vi "Teleop.vi"(10 "Match Info":T1={"Autonomous Elapsed Seconds"=0.0, "TeleOp Elapsed Seconds"=0.0, "Disabled Elapsed Seconds"=0.0, "Visited Autonomous"=FALSE, "Visited TeleOp"=FALSE, "Visited Disabled"=FALSE, "Autonomous Settings"={"Autonomous Style"=enum."Independent", "VI Refnum"=refnum}}, 11 "Call Context":T2) -> ()   [LabVIEW 2020]
doc: "This VI is called for each TeleOp packet received from the DS where the robot is not disabled. It is often used to read from the joysticks and update I/O or to update setpoints for timed control loops. It should complete and return within 20 milliseconds or it may miss DS packets."
uses:
  <vilib>/Rock Robotics/WPI/DriverStation/WPI_DriverStationDerivedRobotMode.ctl
  <vilib>/Rock Robotics/WPI/DriverStation/WPI_DriverStationMatch Info.ctl
  <vilib>/Rock Robotics/WPI/Utilities/WPI_GetSetVariantRefNum.vi
  <vilib>/Rock Robotics/Network Tables/NT Write Boolean Array.vi
  <vilib>/Rock Robotics/Network Tables/NT Write Numeric Array.vi
  <vilib>/Rock Robotics/Network Tables/NT Read Boolean.vi
  <vilib>/Rock Robotics/Network Tables/NT Read Number.vi
  Robot Global Data.vi
panel:
  out "Sample Slider 0":dbl(slide) scale=0.0..5.0
  out "Sample Boolean 1":bool
  out "Sample Boolean 0":bool
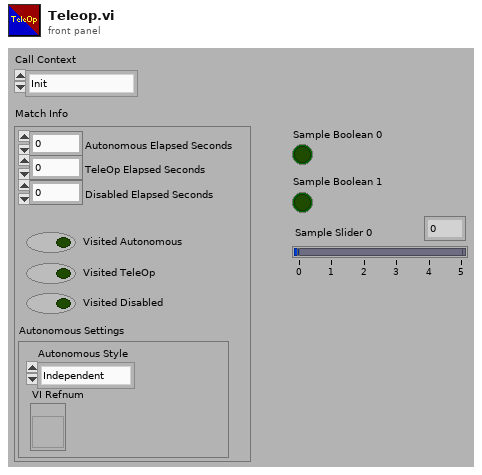
[diagram p1: front panel]
types:
  T1 = typedef "WPI_DriverStationMatch Info.ctl" = cluster{"Autonomous Elapsed Seconds":dbl, "TeleOp Elapsed Seconds":dbl, "Disabled Elapsed Seconds":dbl, "Visited Autonomous":bool, "Visited TeleOp":bool, "Visited Disabled":bool, "Autonomous Settings":cluster{"Autonomous Style":enum16{"Iterative", "Independent"}, "VI Refnum":refnum<vi>}}
  T2 = typedef "WPI_DriverStationDerivedRobotMode.ctl" = enum16{"Init", "Execute", "Stop"}
  T3 = typedef "WPI_JoystickDevRef.ctl" = cluster{"Device":T4}
  T4 = typedef "WPI_JoystickDeviceEnum.ctl" = enum16{"USB 0", "USB 1", "USB 2", "USB 3", "USB 4", "USB 5"}
  T5 = typedef "WPI_RobotDriveDevRef.ctl" = cluster{"DevStatus":errorcluster, "Motors[]":T6[], "Square Inputs":bool, "Max Output":dbl}
  T6 = typedef "WPI_MotorControlDeviceRef.ctl" = cluster{"DeviceStatus":errorcluster, "Type":T7, "PWM":cluster{"PWM Channel":T8, "DeadBand":T9}, "CAN":cluster{"Device Number":u8, "SetOutput VI Ref":variant, "GetOutput VI Ref":variant, "Enable VI Ref":variant, "Disable VI Ref":variant, "Data":variant}, "Invert":bool, "DIO PWM":cluster{"PWM \"Enable\" Channel":T8, "DIOChannel":T10, "PWM Rate":dbl}}
  T7 = typedef "WPI_MotorControlType.ctl" = enum16{"PWM", "CAN", "DIO PWM"}
  T8 = typedef "FPGA_DIOPWMChannel.ctl" = enum8{"PWM 0", "PWM 1", "PWM 2", "PWM 3", "PWM 4", "PWM 5", "PWM 6", "PWM 7", "PWM 8", "PWM 9", "PWM MXP 0", "PWM MXP 1", "PWM MXP 2", "PWM MXP 3", "PWM MXP 4", "PWM MXP 5", "PWM MXP 6", "PWM MXP 7", "PWM MXP 8", "PWM MXP 9", "Invalid"}
  T9 = typedef "WPI_PWMDeadband.ctl" = cluster{"Name":string, "maxPositivePwm":i32, "minPositivePwm":i32, "centerPwm":i32, "maxNegativePwm":i32, "minNegativePwm":i32, "angularRange":u16}
  T10 = typedef "FPGA_DIOChannel.ctl" = enum8{"DIO 0", "DIO 1", "DIO 2", "DIO 3", "DIO 4", "DIO 5", "DIO 6", "DIO 7", "DIO 8", "DIO 9", "DIO MXP 0", "DIO MXP 1", "DIO MXP 2", "DIO MXP 3", "DIO MXP 4", "DIO MXP 5", "DIO MXP 6", "DIO MXP 7", "DIO MXP 8", "DIO MXP 9", "DIO MXP 10", "DIO MXP 11", "DIO MXP 12", "DIO MXP 13", "DIO MXP 14", "DIO MXP 15", "SPI Port CS1", "SPI Port CS2", "SPI Port CS3", "SPI Port MISO", "SPI Port MOSI", "Invalid"}
  T11 = cluster{"Buttons[0]":bool, "Buttons[1]":bool, "Buttons[2]":bool, "Buttons[3]":bool, "Buttons[4]":bool, "Buttons[5]":bool, "Buttons[6]":bool, "Buttons[7]":bool, "Buttons[8]":bool}
  T12 = cluster{"Axes[0]":dbl, "Axes[1]":dbl, "Axes[2]":dbl, "Axes[3]":dbl, "Axes[4]":dbl, "Axes[5]":dbl, "Axes[6]":dbl, "Axes[7]":dbl, "Axes[8]":dbl}
  T13 = typedef "WPI_DigitalOutputDevRef.ctl" = cluster{"DIO Channel":T10, "DevStatus":errorcluster}
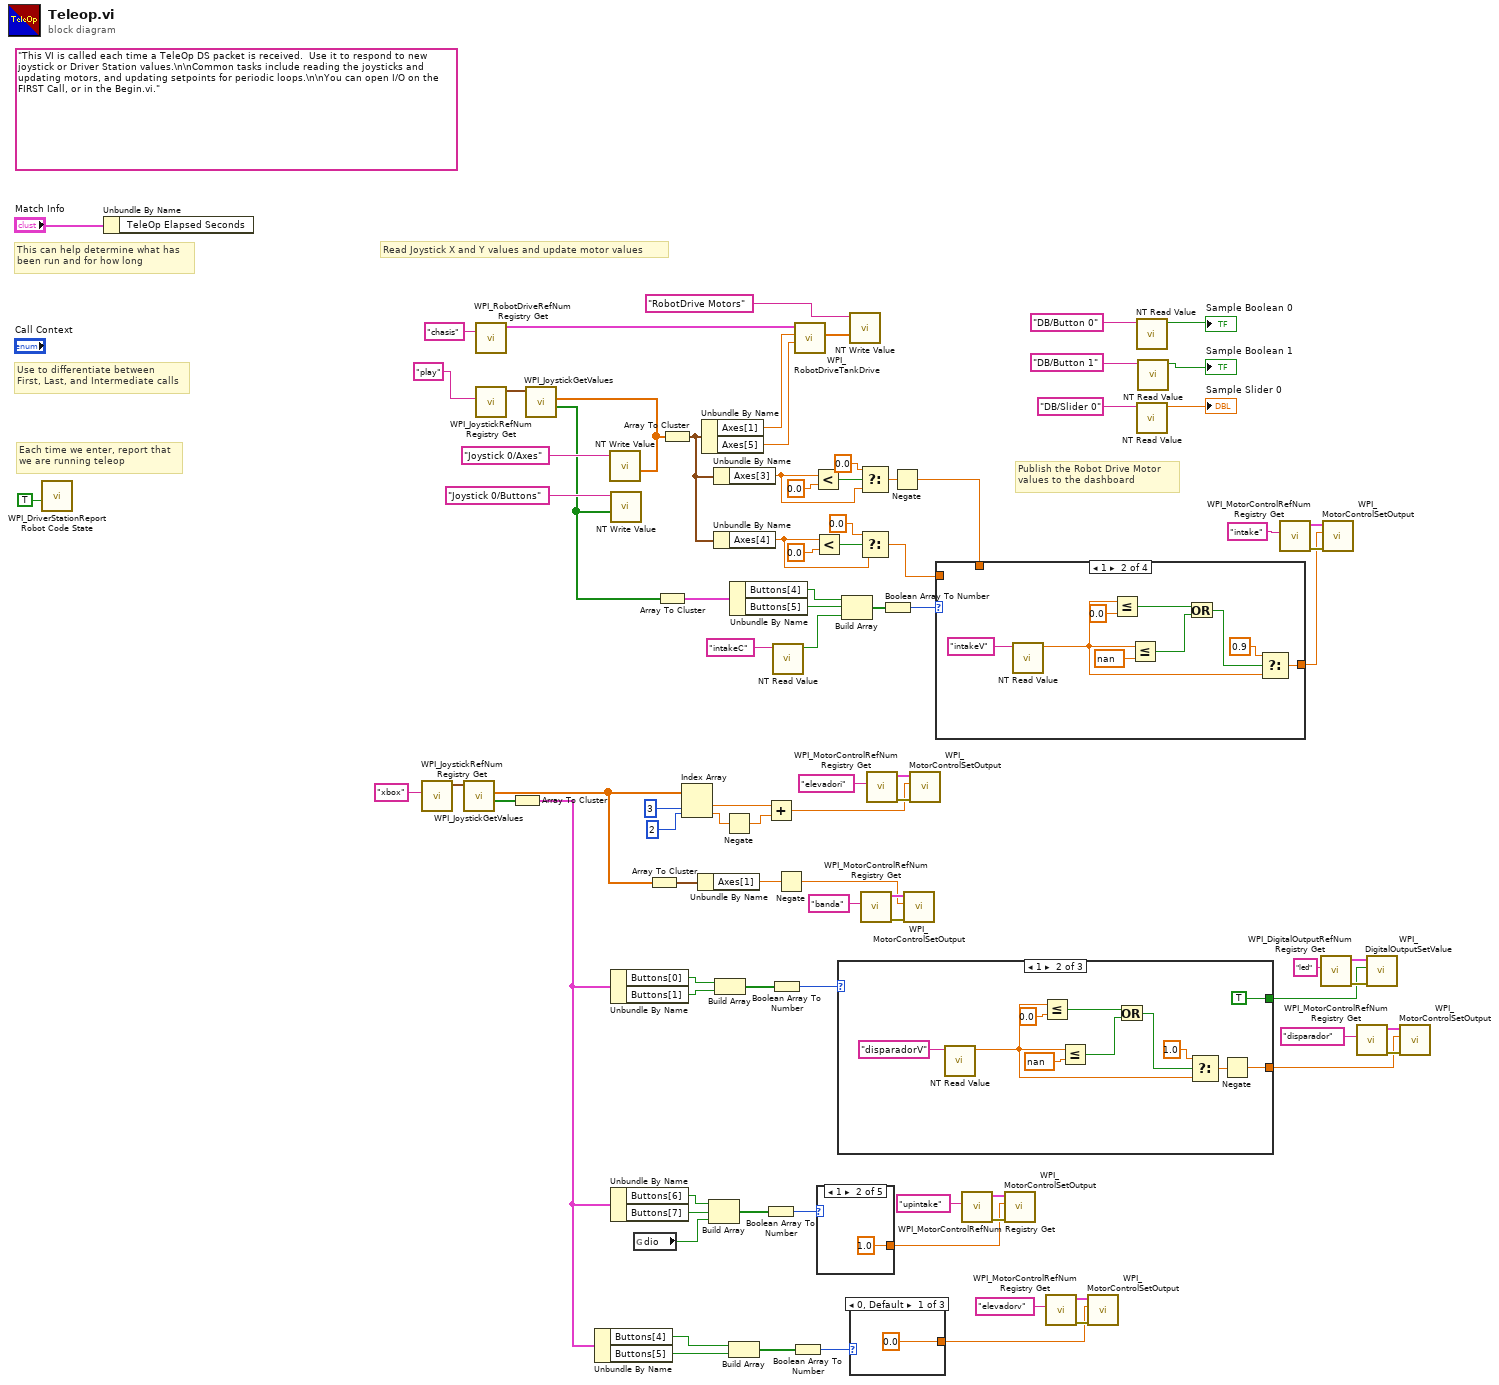
[diagram p0: block diagram]
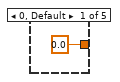
[diagram p2: hidden frame]
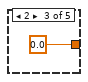
[diagram p3: hidden frame]
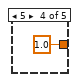
[diagram p4: hidden frame]
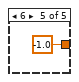
[diagram p5: hidden frame]
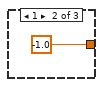
[diagram p6: hidden frame]
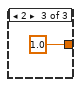
[diagram p7: hidden frame]
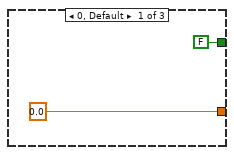
[diagram p8: hidden frame]
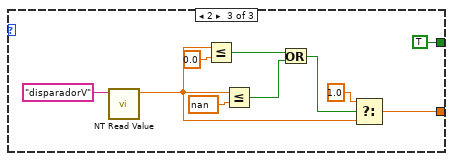
[diagram p9: hidden frame]
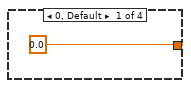
[diagram p10: hidden frame]
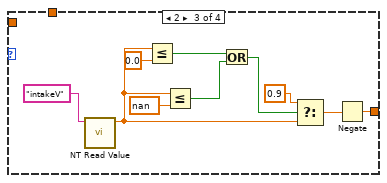
[diagram p11: hidden frame]
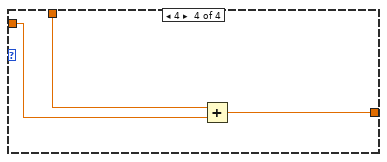
[diagram p12: hidden frame]
diagram:
  (unwired) "This VI is called each time a TeleOp DS packet is received.  Use it to respond to new joystick or Driver Station values.\n\nCommon tasks include reading the joysticks and updating motors, and updating setpoints for periodic loops.\n\nYou can open I/O on the FIRST Call, or in the Begin.vi."
  # "Publish the Robot Drive Motor\nvalues to the dashboard"
  # "Each time we enter, report that\nwe are running teleop"
  # "Use to differentiate between\nFirst, Last, and Intermediate calls"
  # "This can help determine what has\nbeen run and for how long"
  # "Read Joystick X and Y values and update motor values"
  n1 = call <vilib>:"WPI_DriverStationReport Robot Code State.vi"("TeleOp"=TRUE ("Autonomous")) -> ()  [unwired: 10 in, 1 out]
  n2 = Unbundle By Name("Match Info") -> ()  [unwired: 1 out]
  n3 = call <vilib>:"WPI_JoystickRefNum Registry Get.vi"("refnum name"="xbox") -> ("JoystickDevRef"=w73:T3)  [unwired: 1 in, 9 out]
  n4 = call <vilib>:"WPI_JoystickGetValues.vi"("JoystickDevRef"=w73) -> ("Buttons"=w58:bool[], "Axes"=w11:dbl[])  [unwired: 6 in, 3 out]
  n5 = call <vilib>:"WPI_RobotDriveRefNum Registry Get.vi"("refnum name"="chasis") -> ("RobotDriveDevRef"=w90:T5)  [unwired: 1 in, 9 out]
  n6 = call <vilib>:"WPI_JoystickRefNum Registry Get.vi"("refnum name"="play") -> ("JoystickDevRef"=w88:T3)  [unwired: 1 in, 9 out]
  n7 = Array To Cluster(array=w58) -> (cluster=w34:T11)
  n8 = call <vilib>:"WPI_JoystickGetValues.vi"("JoystickDevRef"=w88) -> ("Buttons"=w2:bool[], "Axes"=w37:dbl[])  [unwired: 6 in, 3 out]
  n9 = Unbundle By Name(w34) -> ("Buttons[4]"=w57:bool, "Buttons[5]"=w56:bool)
  n10 = call-poly <vilib>:"NT Write Value.vi"("Numeric Array"=w37, "Name"="Joystick 0/Axes") -> ()  [unwired: 9 in, 1 out]
  n11 = call-poly <vilib>:"NT Write Value.vi"("Boolean Array"=w2, "Name"="Joystick 0/Buttons") -> ()  [unwired: 9 in, 1 out]
  n12 = Unbundle By Name(w34) -> ("Buttons[0]"=w8:bool, "Buttons[1]"=w7:bool)
  n13 = Unbundle By Name(w34) -> ("Buttons[6]"=w48:bool, "Buttons[7]"=w47:bool)
  n14 = global read "Robot Global Data.vi" "dio"() -> (w1:bool)
  n15 = Array To Cluster(array=w11) -> (cluster=w10:T12)
  n16 = Array To Cluster(array=w2) -> (cluster=w12:T11)
  n17 = Array To Cluster(array=w37) -> (cluster=w13:T12)
  n18 = Index Array(array=w11, index #1=3 ("index"), index #2=2 ("index")) -> (element #1=w51:dbl, element #2=w50:dbl)
  n19 = Unbundle By Name(w10) -> ("Axes[1]"=w4:dbl)
  n20 = Unbundle By Name(w13) -> ("Axes[1]"=w36:dbl, "Axes[5]"=w35:dbl)
  n21 = Build Array(w48, w47, w1) -> (w49:bool[])
  n22 = Unbundle By Name(w13) -> ("Axes[3]"=w20:dbl)
  n23 = Unbundle By Name(w13) -> ("Axes[4]"=w15:dbl)
  n24 = Build Array(w8, w7) -> (w9:bool[])
  n25 = Negate(x=w50) -> (-x=w59:dbl)
  n26 = Build Array(w57, w56) -> (w55:bool[])
  n27 = Unbundle By Name(w12) -> ("Buttons[4]"=w29:bool, "Buttons[5]"=w30:bool)
  n28 = Add(x=w51, y=w59) -> (x+y=w24:dbl)
  n29 = Boolean Array To Number(Boolean array=w49) -> (number=w42:u32)
  n30 = Boolean Array To Number(Boolean array=w9) -> (number=w6:u32)
  n31 = call-poly <vilib>:"NT Read Value.vi"("Name"="intakeC") -> ("Boolean"=w31:bool)  [unwired: 9 in, 1 out]
  n32 = Negate(x=w4) -> (-x=w3:dbl)
  n33 = Boolean Array To Number(Boolean array=w55) -> (number=w54:u32)
  n34 = call <vilib>:"WPI_RobotDriveTankDrive.vi"("Right axis value"=w35, "Left axis value"=w36, "RobotDriveDevRef"=w90) -> ("Motor Values"=w78:dbl[])  [unwired: 6 in, 2 out]
  n35 = Less?(x=w20, y=0.0) -> (x < y?=w22:bool)
  n36 = Less?(x=w15, y=0.0) -> (x < y?=w21:bool)
  n37 = case shown="1" w42 {
    tunnel: [0.0 1.0 0.0 1.0 -1.0] -> w43
    frame 0, Default {
    }
    frame 1 {
    }
    frame 2 {
    }
    frame 5 {
    }
    frame 6 {
    }
  }
  n38 = case shown="1" w6 {
    tunnel: [0.0 ("Numeric") w102 w112] -> w69
    tunnel: [FALSE TRUE TRUE] -> w5
    frame 0, Default {
    }
    frame 1 {
      n39 = call-poly <vilib>:"NT Read Value.vi"("Name"="disparadorV") -> ("Numeric"=w104:dbl)  [unwired: 9 in, 1 out]
      n40 = Less Or Equal?(x=w104, y=0.0) -> (x <= y?=w108:bool)
      n41 = Less Or Equal?(x=w104, y=nan) -> (x <= y?=w107:bool)
      n42 = Or(x=w108, y=w107) -> (x .or. y?=w106:bool)
      n43 = Select(t=1.0, s=w106, f=w104) -> (s? t:f=w101:dbl)
      n44 = Negate(x=w101) -> (-x=w102:dbl)
    }
    frame 2 {
      n45 = call-poly <vilib>:"NT Read Value.vi"("Name"="disparadorV") -> ("Numeric"=w114:dbl)  [unwired: 9 in, 1 out]
      n46 = Less Or Equal?(x=w114, y=0.0) -> (x <= y?=w118:bool)
      n47 = Less Or Equal?(x=w114, y=nan) -> (x <= y?=w117:bool)
      n48 = Or(x=w118, y=w117) -> (x .or. y?=w116:bool)
      n49 = Select(t=1.0, s=w116, f=w114) -> (s? t:f=w112:dbl)
    }
  }
  n50 = Build Array(w29, w30, w31) -> (w28:bool[])
  n51 = call-poly <vilib>:"NT Write Value.vi"("Numeric Array"=w78, "Name"="RobotDrive Motors") -> ()  [unwired: 9 in, 1 out]
  n52 = case shown="0, Default" w54 {
    tunnel: [0.0 -1.0 1.0] -> w33
    frame 0, Default {
    }
    frame 1 {
    }
    frame 2 {
    }
  }
  n53 = Select(t=0.0, s=w22, f=w20) -> (s? t:f=w18:dbl)
  n54 = Select(t=0.0, s=w21, f=w15) -> (s? t:f=w16:dbl)
  n55 = call <vilib>:"WPI_MotorControlRefNum Registry Get.vi"("refnum name"="banda") -> ("error out"=w66:errorcluster, "MotorControlDevRef"=w67:T6)  [unwired: 9 in]
  n56 = call <vilib>:"WPI_MotorControlRefNum Registry Get.vi"("refnum name"="elevadori") -> ("error out"=w63:errorcluster, "MotorControlDevRef"=w64:T6)  [unwired: 9 in]
  n57 = Boolean Array To Number(Boolean array=w28) -> (number=w27:u32)
  n58 = Negate(x=w18) -> (-x=w17:dbl)
  n59 = call <vilib>:"WPI_MotorControlSetOutput.vi"("error in (no error)"=w66, "Output"=w3, "MotorControlDevRef"=w67) -> ()  [unwired: 6 in, 3 out]
  n60 = call <vilib>:"WPI_MotorControlSetOutput.vi"("error in (no error)"=w63, "Output"=w24, "MotorControlDevRef"=w64) -> ()  [unwired: 6 in, 3 out]
  n61 = case shown="1" w27 {
    tunnel: [0.0 w125 w134 w146] -> w26
    tunnel: w16 -> [_ _ _ w144]
    tunnel: w17 -> [_ _ _ w145]
    frame 0, Default {
    }
    frame 1 {
      n62 = call-poly <vilib>:"NT Read Value.vi"("Name"="intakeV") -> ("Numeric"=w133:dbl)  [unwired: 9 in, 1 out]
      n63 = Less Or Equal?(x=w133, y=0.0) -> (x <= y?=w130:bool)
      n64 = Less Or Equal?(x=w133, y=nan) -> (x <= y?=w131:bool)
      n65 = Or(x=w130, y=w131) -> (x .or. y?=w132:bool)
      n66 = Select(t=0.9, s=w132, f=w133) -> (s? t:f=w125:dbl)
    }
    frame 2 {
      n67 = call-poly <vilib>:"NT Read Value.vi"("Name"="intakeV") -> ("Numeric"=w142:dbl)  [unwired: 9 in, 1 out]
      n68 = Less Or Equal?(x=w142, y=0.0) -> (x <= y?=w139:bool)
      n69 = Less Or Equal?(x=w142, y=nan) -> (x <= y?=w140:bool)
      n70 = Or(x=w139, y=w140) -> (x .or. y?=w141:bool)
      n71 = Select(t=0.9, s=w141, f=w142) -> (s? t:f=w143:dbl)
      n72 = Negate(x=w143) -> (-x=w134:dbl)
    }
    frame 4 {
      n73 = Add(x=w145, y=w144) -> (x+y=w146:dbl)
    }
  }
  n74 = call <vilib>:"WPI_MotorControlRefNum Registry Get.vi"("refnum name"="upintake") -> ("error out"=w44:errorcluster, "MotorControlDevRef"=w45:T6)  [unwired: 9 in]
  n75 = call <vilib>:"WPI_MotorControlSetOutput.vi"("error in (no error)"=w44, "Output"=w43, "MotorControlDevRef"=w45) -> ()  [unwired: 6 in, 3 out]
  n76 = call <vilib>:"WPI_MotorControlRefNum Registry Get.vi"("refnum name"="elevadorv") -> ("error out"=w60:errorcluster, "MotorControlDevRef"=w61:T6)  [unwired: 9 in]
  n77 = call <vilib>:"WPI_MotorControlSetOutput.vi"("error in (no error)"=w60, "Output"=w33, "MotorControlDevRef"=w61) -> ()  [unwired: 6 in, 3 out]
  n78 = call-poly <vilib>:"NT Read Value.vi"("Name"="DB/Button 0" ("refnum name")) -> ("Boolean"=→"Sample Boolean 0":bool)  [unwired: 9 in, 1 out]
  n79 = call-poly <vilib>:"NT Read Value.vi"("Name"="DB/Slider 0" ("refnum name")) -> ("Numeric"=→"Sample Slider 0":dbl)  [unwired: 9 in, 1 out]
  n80 = call-poly <vilib>:"NT Read Value.vi"("Name"="DB/Button 1" ("refnum name")) -> ("Boolean"=→"Sample Boolean 1":bool)  [unwired: 9 in, 1 out]
  n81 = call <vilib>:"WPI_MotorControlRefNum Registry Get.vi"("refnum name"="intake") -> ("error out"=w75:errorcluster, "MotorControlDevRef"=w76:T6)  [unwired: 9 in]
  n82 = call <vilib>:"WPI_DigitalOutputRefNum Registry Get.vi"("refnum name"="led") -> ("error out"=w40:errorcluster, "DigitalOutputDevRef"=w39:T13)  [unwired: 9 in]
  n83 = call <vilib>:"WPI_MotorControlSetOutput.vi"("error in (no error)"=w75, "Output"=w26, "MotorControlDevRef"=w76) -> ()  [unwired: 6 in, 3 out]
  n84 = call <vilib>:"WPI_MotorControlRefNum Registry Get.vi"("refnum name"="disparador") -> ("error out"=w70:errorcluster, "MotorControlDevRef"=w71:T6)  [unwired: 9 in]
  n85 = call <vilib>:"WPI_DigitalOutputSetValue.vi"("error in (no error)"=w40, "Value"=w5, "DigitalOutputDevRef"=w39) -> ()  [unwired: 7 in, 2 out]
  n86 = call <vilib>:"WPI_MotorControlSetOutput.vi"("error in (no error)"=w70, "Output"=w69, "MotorControlDevRef"=w71) -> ()  [unwired: 6 in, 3 out]
